vi "solar_voy_def Parse Args (Label).vi"(11 "Default ITEM":T1) -> (3 "ITEM out":T1)   [LabVIEW 2018]
doc: "This parses a parameters label by item arguments.\n\n<b>Arguments:</b>\nt=TYPE (block|string|int|uint|float) - Sets the COSMOS data type\nlv=LVTYPE (u8..dbl,str,bool,etc.) - Sets the LabVIEW data type\nb=BIT_SIZE - Sets the total parameter|item bit size\ne=EACH_BIT_SIZE - Sets the element bit size for string or block arrays only\ns=STATE|STATE - Sets the states starting at value 0:STATE|1:STATE|etc.\nid - Sets the ID flag\n\nExamples: \nMYBLOCKARRAY,t=block,lv=string,b=64,e=16 # 1D array of U16 blocks of 4 elements (64 bits / 16 each) \nMYU16KEY,t=uint,lv=u16,b=16,id # U16 id parameter\nMYBOOLEAN,t=uint,lv=boolean,b=1,s=OK|ERROR # 1 bit boolean with false:OK, true:ERROR states"
uses:
  solar_voy_def_ctl MODIFIERS STATE.ctl
  solar_voy_def_ctl MODIFIERS CONVERSION.ctl
  solar_voy_def_ctl MODIFIERS UNITS.ctl
  solar_voy_def_ctl MODIFIERS LIMITS.ctl
  solar_voy_def_ctl MODIFIERS.ctl
  solar_voy_def_ctl ITEM TYPE.ctl
  type/solar_type Item Type.ctl
  solar_voy_def_ctl ITEM.ctl
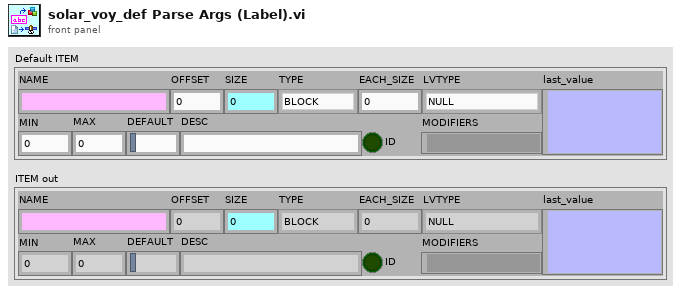
[diagram p1: front panel]
types:
  T1 = typedef "solar_voy_def_ctl ITEM.ctl" = cluster{"NAME":string, "OFFSET":i32, "SIZE":i32, "TYPE":T2, "EACH_SIZE":i32, "LVTYPE":T3, "MIN":dbl, "MAX":dbl, "DEFAULT":string, "DESC":string, "ID":bool, "MODIFIERS":variant, "last_value":variant}
  T2 = typedef "solar_voy_def_ctl ITEM TYPE.ctl" = enum8{"BLOCK", "INT", "UINT", "FLOAT", "STRING"}
  T3 = typedef "solar_type Item Type.ctl" = enum16{"NULL", "UNKNOWN", "CLUSTER", "I8", "I16", "I32", "I64", "U8", "U16", "U32", "U64", "U8_ENUM", "U16_ENUM", "U32_ENUM", "SGL", "DBL", "BOOLEAN", "STRING", "PATH", "VISA", "TAG", "TIME", "I8_1D", "I16_1D", "I32_1D", "I64_1D", "U8_1D", "U16_1D", "U32_1D", "U64_1D", "U8_ENUM_1D", "U16_ENUM_1D", "U32_ENUM_1D", "SGL_1D", "DBL_1D", "BOOLEAN_1D", "STRING_1D", "PATH_1D", "VISA_1D", "TAG_1D", "TIME_1D", "I8_2D", "I16_2D", "I32_2D", "I64_2D", "U8_2D", "U16_2D", "U32_2D", "U64_2D", "U8_ENUM_2D", "U16_ENUM_2D", "U32_ENUM_2D", "SGL_2D", "DBL_2D", "BOOLEAN_2D", "STRING_2D", "PATH_2D", "VISA_2D", "TAG_2D", "TIME_2D"}
  T4 = typedef "solar_voy_def_ctl MODIFIERS STATE.ctl" = cluster{"KEY":string, "VALUE":string, "COLOR":string, "DESC":string, "HZRD":bool}
  T5 = typedef "solar_voy_def_ctl MODIFIERS.ctl" = cluster{"LIMITS":T6, "UNITS":T7, "STATES":T4[], "CONVERSION":T8, "FORMAT":string, "REQUIRED":bool, "META":string[][]}
  T6 = typedef "solar_voy_def_ctl MODIFIERS LIMITS.ctl" = cluster{"NAME":string, "PERSIST":i32, "EN":bool, "RED_LO":dbl, "YEL_LO":dbl, "YEL_HI":dbl, "RED_HI":dbl, "GRN_LO":dbl, "GRN_HI":dbl, "FILENAME":string, "ARGS":string}
  T7 = typedef "solar_voy_def_ctl MODIFIERS UNITS.ctl" = cluster{"FULL":string, "ABV":string}
  T8 = typedef "solar_voy_def_ctl MODIFIERS CONVERSION.ctl" = cluster{"GENERIC":string, "FILENAME":string, "ARGS":string, "POLYS":cluster{"SEG":bool, "POLY":dbl[]}[]}
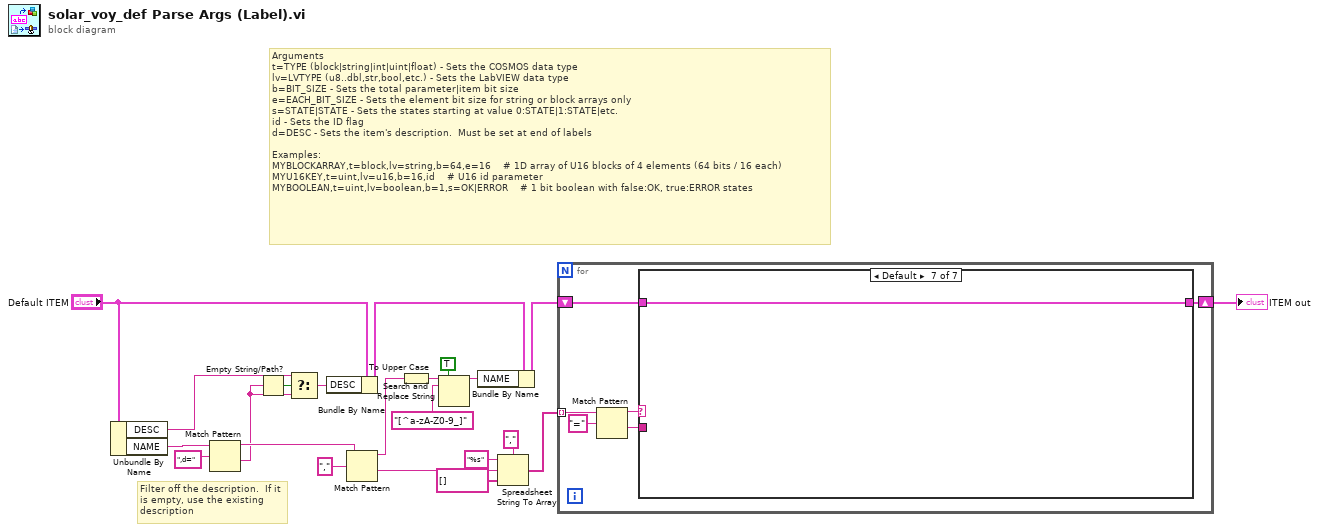
[diagram p0: block diagram]
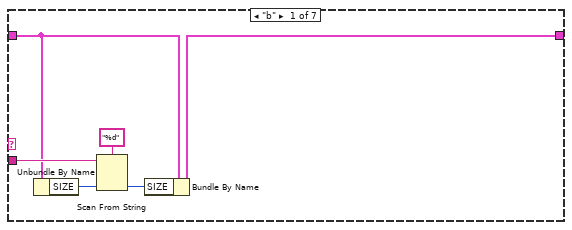
[diagram p2: hidden frame]
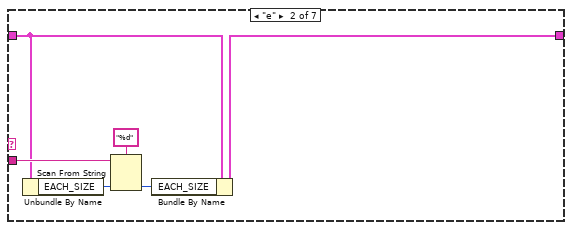
[diagram p3: hidden frame]
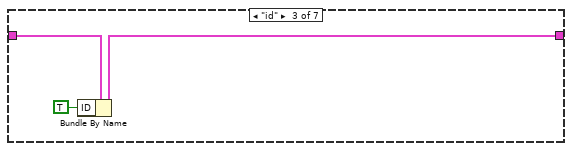
[diagram p4: hidden frame]
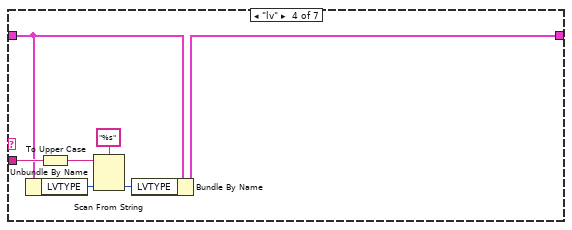
[diagram p5: hidden frame]
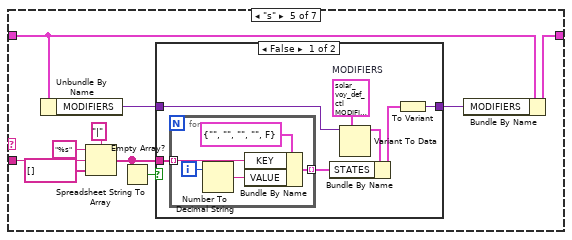
[diagram p6: hidden frame]
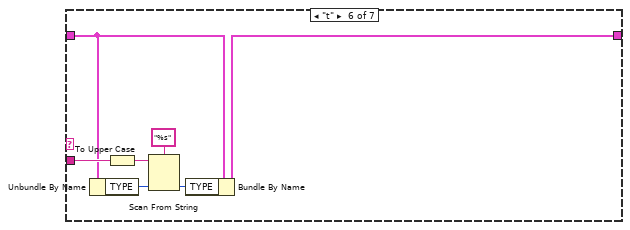
[diagram p8: hidden frame]
diagram:
  # "Filter off the description.  If it is empty, use the existing description"
  # "Arguments\nt=TYPE (block|string|int|uint|float) - Sets the COSMOS data type\nlv=LVTYPE (u8..dbl,str,bool,etc.) - Sets the LabVIEW data type\nb=BIT_SIZE - Sets the total parameter|item bit size\ne=EACH_BIT_SIZE - Sets the element bit size for string or block arrays only\ns=STATE|STATE - Sets the states starting at value 0:STATE|1:STATE|etc.\nid - Sets the ID flag\nd=DESC - Sets the item's description.  Must be set at end of labels \n\nExamples: \nMYBLOCKARRAY,t=block,lv=string,b=64,e=16    # 1D array of U16 blocks of 4 elements (64 bits / 16 each) \nMYU16KEY,t=uint,lv=u16,b=16,id    # U16 id parameter\nMYBOOLEAN,t=uint,lv=boolean,b=1,s=OK|ERROR    # 1 bit boolean with false:OK, true:ERROR states"
  n1 = Unbundle By Name("Default ITEM") -> ("DESC"=w2:string, "NAME"=w7:string)
  n2 = Match Pattern(string=w7, regular expression=",d=") -> (before substring=w6:string, after substring=w3:string)  [unwired: 1 in, 2 out]
  n3 = Empty String/Path?(string/path=w3) -> (empty?=w4:bool)
  n4 = Select(t=w2, s=w4, f=w3) -> (s? t:f=w1:string)
  n5 = Bundle By Name(cluster="Default ITEM", "DESC"=w1) -> (w5:T1)
  n6 = Match Pattern(string=w6, regular expression=",") -> (before substring=w18:string, after substring=w17:string)  [unwired: 1 in, 2 out]
  n7 = To Upper Case(1:w18) -> (0:w19:string)
  n8 = Search and Replace String(replace all?=TRUE, input string=w19, search string="[^a-zA-Z0-9_]") -> (result string=w9:string)  [unwired: 5 in, 3 out]
  n9 = Bundle By Name(cluster=w5, "NAME"=w9) -> (w10:T1)
  n10 = Spreadsheet String To Array(delimiter (Tab)=",", format string="%s", spreadsheet string=w17, array type (2D Dbl)=string[] []) -> (array=w13:string[])
  n11 = for {
    tunnel: w13 -> [w28] mode=indexing
    shift-right: [w25] -> w12
    shift-left: w10 -> [w24]
    n12 = Match Pattern(string=w28, regular expression="=") -> (before substring=w26:string, after substring=w23:string)  [unwired: 1 in, 2 out]
    n13 = case shown="Default" w26 {
      tunnel: [w30 w36 w42 w46 w59 w76 w81] -> w25
      tunnel: w24 -> [w33 w39 w43 w49 w60 w79 w81]
      tunnel: w23 -> [w34 w40 _ w50 w55 w80 _]
      frame "b" {
        n14 = Unbundle By Name(w33) -> ("SIZE"=w32:i32)
        n15 = Scan From String(format string="%d", input string=w34, default 1=w32) -> (output 1=w29:i32)  [unwired: 2 in, 3 out]
        n16 = Bundle By Name(cluster=w33, "SIZE"=w29) -> (w30:T1)
      }
      frame "e" {
        n17 = Unbundle By Name(w39) -> ("EACH_SIZE"=w38:i32)
        n18 = Scan From String(format string="%d", input string=w40, default 1=w38) -> (output 1=w35:i32)  [unwired: 2 in, 3 out]
        n19 = Bundle By Name(cluster=w39, "EACH_SIZE"=w35) -> (w36:T1)
      }
      frame "id" {
        n20 = Bundle By Name(cluster=w43, "ID"=TRUE) -> (w42:T1)
      }
      frame "lv" {
        n21 = Unbundle By Name(w49) -> ("LVTYPE"=w48:T3)
        n22 = To Upper Case(1:w50) -> (0:w44:string)
        n23 = Scan From String(format string="%s", input string=w44, default 1=w48) -> (output 1=w45:T3)  [unwired: 2 in, 3 out]
        n24 = Bundle By Name(cluster=w49, "LVTYPE"=w45) -> (w46:T1)
      }
      frame "s" {
        n25 = Unbundle By Name(w60) -> ("MODIFIERS"=w51:variant)
        n26 = Spreadsheet String To Array(delimiter (Tab)="|", format string="%s", spreadsheet string=w55, array type (2D Dbl)=string[] []) -> (array=w53:string[])
        n27 = Empty Array?(array=w53) -> (empty?=w52:bool)
        n28 = case shown="False" w52 {
          tunnel: [w61 w73] -> w54
          tunnel: w53 -> [w67 _]
          tunnel: w51 -> [w63 w73]
          frame False {
            w64 = T5 {"LIMITS"={"NAME"="", "PERSIST"=0, "EN"=FALSE, "RED_LO"=0.0, "YEL_LO"=0.0, "YEL_HI"=0.0, "RED_HI"=0.0, "GRN_LO"=0.0, "GRN_HI"=0.0, "FILENAME"="", "ARGS"=""}, "UNITS"={"FULL"="", "ABV"=""}, "STATES"=[], "CONVERSION"={"GENERIC"="", "FILENAME"="", "ARGS"="", "POLYS"=[]}, "FORMAT"="", "REQUIRED"=FALSE, "META"=[]}  # MODIFIERS
            n29 = for {
              tunnel: w67 -> [w70] mode=indexing
              tunnel: [w68] -> w66 mode=indexing
              i -> [w72]
              n30 = Number To Decimal String(number=w72) -> (decimal integer string=w69:string)  [unwired: 1 in]
              n31 = Bundle By Name(cluster=T4 {"KEY"="", "VALUE"="", "COLOR"="", "DESC"="", "HZRD"=FALSE} ("STATE"), "KEY"=w70, "VALUE"=w69) -> (w68:T4)
            }
            n32 = Variant To Data(type=w64, Variant=w63) -> (data=w62:T5)  [unwired: 1 in, 1 out]
            n33 = Bundle By Name(cluster=w62, "STATES"=w66) -> (w65:T5)
            n34 = To Variant(anything=w65) -> (Variant=w61:variant)
          }
          frame True {
          }
        }
        n35 = Bundle By Name(cluster=w60, "MODIFIERS"=w54) -> (w59:T1)
      }
      frame "t" {
        n36 = Unbundle By Name(w79) -> ("TYPE"=w78:T2)
        n37 = To Upper Case(1:w80) -> (0:w74:string)
        n38 = Scan From String(format string="%s", input string=w74, default 1=w78) -> (output 1=w75:T2)  [unwired: 2 in, 3 out]
        n39 = Bundle By Name(cluster=w79, "TYPE"=w75) -> (w76:T1)
      }
      frame Default {
      }
    }
  }
  "ITEM out" <- w12
